vi "Check for Trigger.vi"(2 "# Data Points":i32, 3 "Current Values":dbl[](array[numeric]) format="%.2e", 4 "Trigger Column":u32, 5 "Æ Trigger Value":dbl format="%.2f") -> (0 "# Data Points Out":i32, 1 "Wait":bool)   [LabVIEW 2025]
doc: "Decides if the inputs have changed by an amount greater than delta so that a reading is triggered (saved).\nScott Hannahs, FBNML, Jan 1992\nAuthor: Scott Hannahs <sth@magnet.fsu.edu>\n\nThis software is licensed for use under the “MIT License\"\nCopyright (c) 2025 Scott Hannahs, sth@sth@magnet.sthnet.net\n\nPermission is hereby granted, free of charge, to any person obtaining a copy of this software and associated documentation files (the \"Software\"), to deal in the Software without restriction, including without limitation the rights to use, copy, modify, merge, publish, distribute, sublicense, and/or sell copies of the Software, and to permit persons to whom the Software is furnished to do so, subject to the following conditions: The above copyright notice and this permission notice shall be included in all copies or substantial portions of the Software.\n\nTHE SOFTWARE IS PROVIDED \"AS IS\", WITHOUT WARRANTY OF ANY KIND, EXPRESS OR IMPLIED, INCLUDING BUT NOT LIMITED TO THE WARRANTIES OF MERCHANTABILITY, FITNESS FOR A PARTICULAR PURPOSE AND NONINFRINGEMENT. IN NO EVENT SHALL THE AUTHORS OR COPYRIGHT HOLDERS BE LIABLE FOR ANY CLAIM, DAMAGES OR OTHER LIABILITY, WHETHER IN AN ACTION OF CONTRACT, TORT OR OTHERWISE, ARISING FROM, OUT OF OR IN CONNECTION WITH THE SOFTWARE OR THE USE OR OTHER DEALINGS IN THE SOFTWARE."
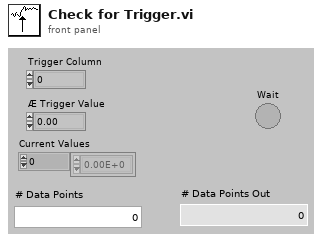
[diagram p1: front panel]
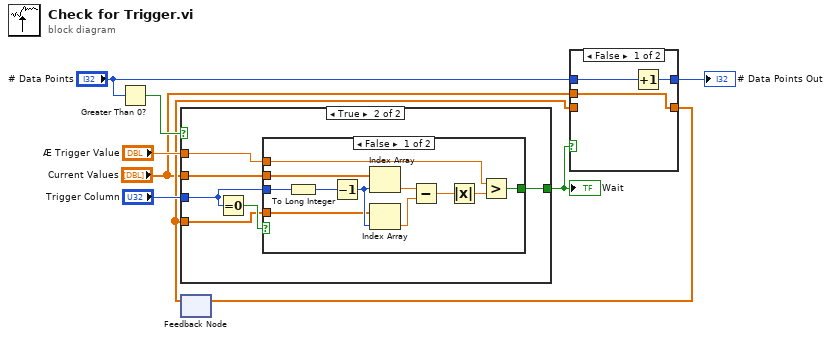
[diagram p0: block diagram]
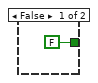
[diagram p3: hidden frame]
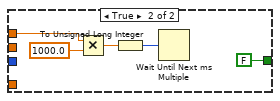
[diagram p4: hidden frame]
diagram:
  n1 = Greater Than 0?(x="# Data Points") -> (x > 0?=w7:bool)
  n2 = feedback #1() -> (w2:dbl[])  [unwired: 1 in]
  n3 = case shown="True" w7 {
    tunnel: "Trigger Column" -> [_ w15]
    tunnel: "Æ Trigger Value" -> [_ w14]
    tunnel: [FALSE w13] -> w4
    tunnel: "Current Values" -> [_ w12]
    tunnel: w2 -> [_ w11]
    frame False {
    }
    frame True {
      n4 = Equal To 0?(x=w15) -> (x = 0?=w16:bool)
      n5 = case shown="False" w16 {
        tunnel: [w23 FALSE] -> w13
        tunnel: w14 -> [w26 w30]
        tunnel: w15 -> [w27 _]
        tunnel: w12 -> [w19 _]
        tunnel: w11 -> [w18 _]
        frame False {
          n6 = To Long Integer(number=w27) -> (32bit integer=w17:i32)
          n7 = Decrement(x=w17) -> (x-1=w21:i32)
          n8 = Index Array(array=w19, index=w21) -> (element=w22:dbl)
          n9 = Index Array(array=w18, index=w21) -> (element=w20:dbl)
          n10 = Subtract(x=w22, y=w20) -> (x-y=w25:dbl)
          n11 = Absolute Value(x=w25) -> (abs(x)=w24:dbl)
          n12 = Greater?(x=w26, y=w24) -> (0:w23:bool)
        }
        frame True {
          n13 = Multiply(x=w30, y=1000.0) -> (x*y=w29:dbl)
          n14 = To Unsigned Long Integer(number=w29) -> (unsigned 32bit integer=w28:u32)
          n15 = Wait Until Next ms Multiple(millisecond multiple=w28) -> ()  [unwired: 1 out]
        }
      }
    }
  }
  "Wait" <- w4
  n16 = case shown="False" w4 {
    tunnel: [w34 w37] -> w5
    tunnel: "# Data Points" -> [w35 w37]
    tunnel: [w33 w36] -> w3
    tunnel: w2 -> [_ w36]
    tunnel: "Current Values" -> [w33 _]
    frame False {
      n17 = Increment(x=w35) -> (x+1=w34:i32)
    }
    frame True {
    }
  }
  "# Data Points Out" <- w5
  n18 = feedback-in #1(w3) -> ()
